vi "New Layout.vi"(8 "Error In":errorcluster, 9 "StatusBar":refnum<class "StatusBar.lvclass">, 10 "SideMenu":refnum<class "SideMenu.lvclass">, 11 "TitleBar":refnum<class "TitleBar.lvclass">) -> (0 "Error Out":errorcluster, 3 "Layout":refnum<class "Layout.lvclass">)   [LabVIEW 2021, in "Appearance Actor.lvlib" / "Layout.lvclass"]
uses:
  Layout.lvclass
  Layout Components/SideMenus/SideMenu/SideMenu.lvclass
  Layout Components/StatusBars/StatusBar/StatusBar.lvclass
  Layout Components/TitleBars/TitleBar/TitleBar.lvclass
  Layout.lvclass/Layout.ctl
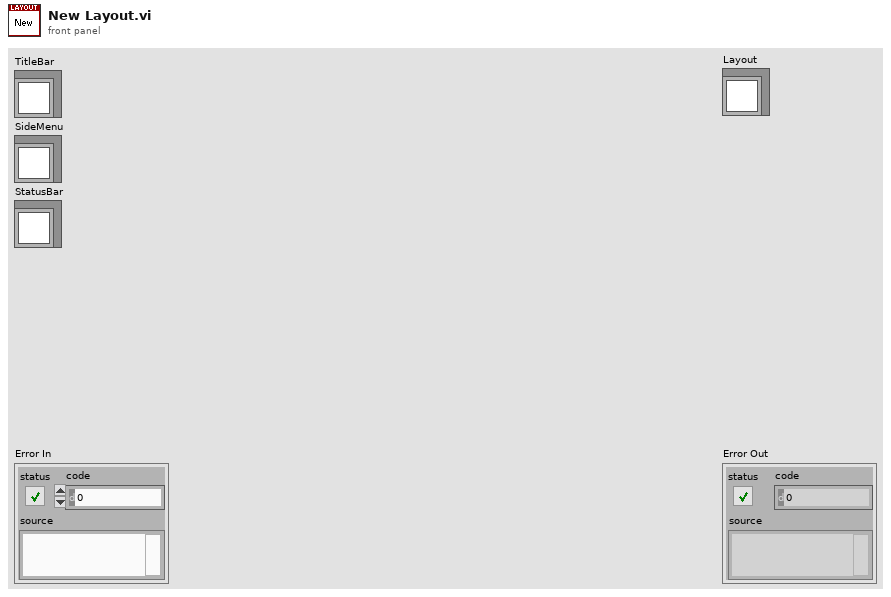
[diagram p1: front panel]
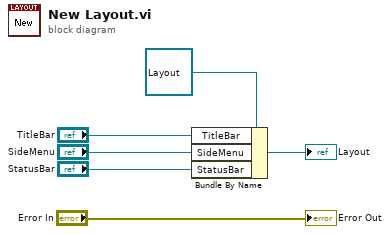
[diagram p0: block diagram]
diagram:
  n1 = Bundle By Name(cluster=refnum<class "Layout.lvclass"> refnum ("Layout"), "TitleBar"="TitleBar", "SideMenu"="SideMenu", "StatusBar"="StatusBar") -> (→"Layout":refnum<class "Layout.lvclass">)
  "Error Out" <- "Error In"
